vi "noise.vi"() -> ()   [LabVIEW 2009]
uses:
  <vilib>/Analysis/NI_AALBase.lvlib
panel:
  out "歪み率":dbl
  out "出力":cluster{dbl[], dbl[]}(graph) caption="XYグラフ"
  out "送信波":cluster{dbl[], dbl[]}(graph)
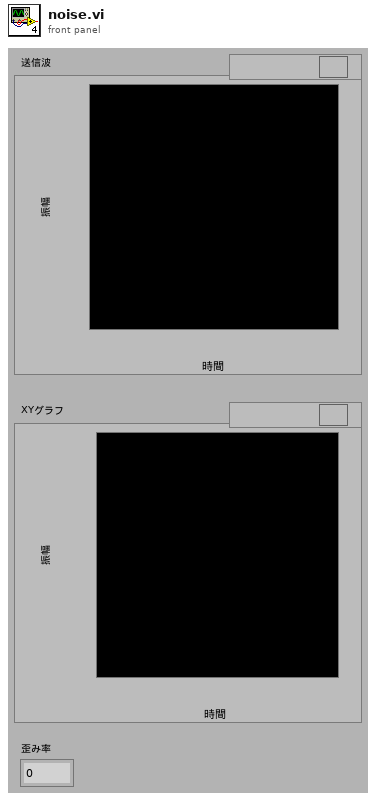
[diagram p1: front panel]
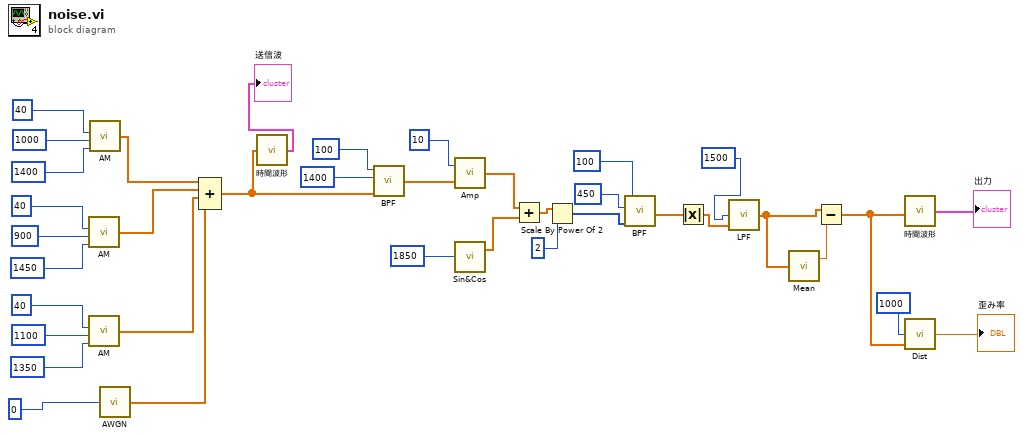
[diagram p0: block diagram]
diagram:
  n1 = call "AM.vi"("変調度 [%]"=40, "変調周波数 [Hz]"=900, "搬送波周波数 [kHz]"=1450) -> ("変調波"=w27:dbl[])  [unwired: 2 in]
  n2 = call "AM.vi"("変調度 [%]"=40, "変調周波数 [Hz]"=1100, "搬送波周波数 [kHz]"=1350) -> ("変調波"=w26:dbl[])  [unwired: 2 in]
  n3 = call "AM.vi"("変調度 [%]"=40, "変調周波数 [Hz]"=1000, "搬送波周波数 [kHz]"=1400) -> ("変調波"=w28:dbl[])  [unwired: 2 in]
  n4 = call "AWGN.vi"("振幅値"=0) -> ("出力"=w25:dbl[])
  n5 = Compound Arithmetic op=ADD(w28, w27, w26, w25) -> (w22:dbl[])
  n6 = call "時間波形.vi"("入力"=w22) -> ("時間波形"=→"送信波":cluster{dbl[], dbl[]})
  n7 = call "BPF.vi"("X"=w22, "中心周波数 [kHz]"=1400, "Q"=100) -> ("BPF出力"=w20:dbl[])  [unwired: 1 in]
  n8 = call "Amp.vi"("入力"=w20, "増幅率"=10) -> ("出力"=w15:dbl[])
  n9 = call "Sin&Cos.vi"("周波数[kHz]"=1850) -> ("sin"=w14:dbl[])  [unwired: 1 out]
  n10 = Add(x=w15, y=w14) -> (x+y=w17:dbl[])
  n11 = Scale By Power Of 2(n=w17, x=2) -> (x*2^n=w13:i32[])
  n12 = call "BPF.vi"("X"=w13, "中心周波数 [kHz]"=450, "Q"=100) -> ("BPF出力"=w7:dbl[])  [unwired: 1 in]
  n13 = Absolute Value(x=w7) -> (abs(x)=w6:dbl[])
  n14 = call "LPF.vi"("入力"=w6, "カットオフ周波数 [Hz]"=1500) -> ("LPF出力"=w4:dbl[])  [unwired: 1 in]
  n15 = call <vilib>:"Mean.vi"("X"=w4) -> ("mean"=w5:dbl)  [unwired: 1 out]
  n16 = Subtract(x=w4, y=w5) -> (x-y=w3:dbl[])
  n17 = call "時間波形.vi"("入力"=w3) -> ("時間波形"=→"出力":cluster{dbl[], dbl[]})
  n18 = call "Dist.vi"("入力"=w3, "基本周波数 [Hz]"=1000) -> ("ひずみ率"=→"歪み率":dbl)  [unwired: 1 in]
